vi "solar_tcp Open.vi"(6 "Suppress Errors? (T)":bool=TRUE, 8 "error in (no error)":errorcluster, 11 "Config":T1={"TCPServer"=enum."SERVER", "ServerPort"=0, "IPAddress"="", "ClientPort"=0, "HdrSizeBytes"=4, "HdrLenSubtractBytes"=4, "HdrLenOffsetBits"=0, "HdrLenSizeBits"=32}) -> (0 "error out":errorcluster, 1 "Connected":bool, 3 "TCP Data out":T2 {"Debug"."Time" format="%<%Y-%m-%d\n%H:%M:%S%3u>T"})   [LabVIEW 2018]
doc: "This opens a TCP connection specified by <b>Config</b> options."
uses:
  solar_tcp_ctl Action.ctl
  solar_tcp_ctl Config.ctl
  solar_tcp_ctl Debug.ctl
  solar_tcp_ctl Data.ctl
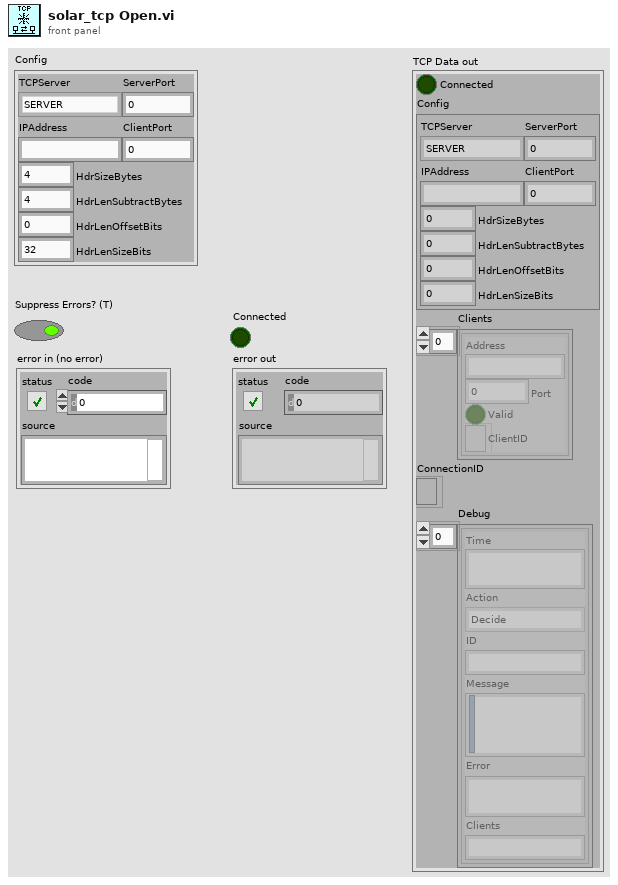
[diagram p1: front panel]
types:
  T1 = typedef "solar_tcp_ctl Config.ctl" = cluster{"TCPServer":enum8{"SERVER", "CLIENT"}, "ServerPort":u16, "IPAddress":string, "ClientPort":u16, "HdrSizeBytes":i32, "HdrLenSubtractBytes":i32, "HdrLenOffsetBits":i32, "HdrLenSizeBits":i32}
  T2 = typedef "solar_tcp_ctl Data.ctl" = cluster{"Connected":bool, "Config":T1, "Clients":cluster{"Address":string, "Port":u16, "Valid":bool, "ClientID":refnum<k5>}[], "ConnectionID":refnum<k5>, "Debug":T3[]}
  T3 = typedef "solar_tcp_ctl Debug.ctl" = cluster{"Time":timestamp, "Action":T4, "ID":string, "Message":string, "Error":string, "Clients":string}
  T4 = typedef "solar_tcp_ctl Action.ctl" = enum16{"Decide", "CreateListener", "Open", "Read", "Write", "Close", "Shutdown", "Done", "ChangePort"}
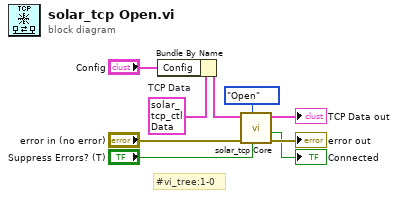
[diagram p0: block diagram]
diagram:
  w3 = T2 {"Connected"=FALSE, "Config"={"TCPServer"=enum."SERVER", "ServerPort"=0, "IPAddress"="", "ClientPort"=0, "HdrSizeBytes"=4, "HdrLenSubtractBytes"=0, "HdrLenOffsetBits"=0, "HdrLenSizeBits"=32}, "Clients"=[], "ConnectionID"=refnum, "Debug"=[]}  # TCP Data
  # "#vi_tree:1-0"
  n1 = Bundle By Name(cluster=w3, "Config"="Config") -> (w2:T2)
  n2 = call "solar_tcp Core.vi"("Suppress Errors? (T)"="Suppress Errors? (T)", "Action"=solar_tcp_ctl_Action."Open", "error in (no error)"="error in (no error)", "TCP Data in"=w2) -> ("error out"=→"error out":errorcluster, "Connected"=→"Connected":bool, "TCP Data out"=→"TCP Data out":T2)  [unwired: 4 in, 1 out]
